vi "Inline Temporary SubVIs.vi"(8 "error in (no error)":errorcluster, 11 "Responsive Mock Class Generator in":refnum<class "Responsive Mock Class Generator.lvclass">) -> (0 "error out":errorcluster, 3 "Responsive Mock Class Generator out":refnum<class "Responsive Mock Class Generator.lvclass">)   [LabVIEW 2020, in "Responsive Mock Class Generator.lvclass"]
uses:
  Responsive Mock Class Generator.lvclass
  Responsive Mock Class Generator.lvclass/Responsive Mock Class Generator.ctl
  Framework/Responsive Mock/Append Control Value.vi
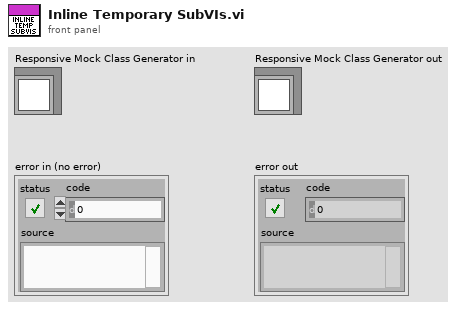
[diagram p1: front panel]
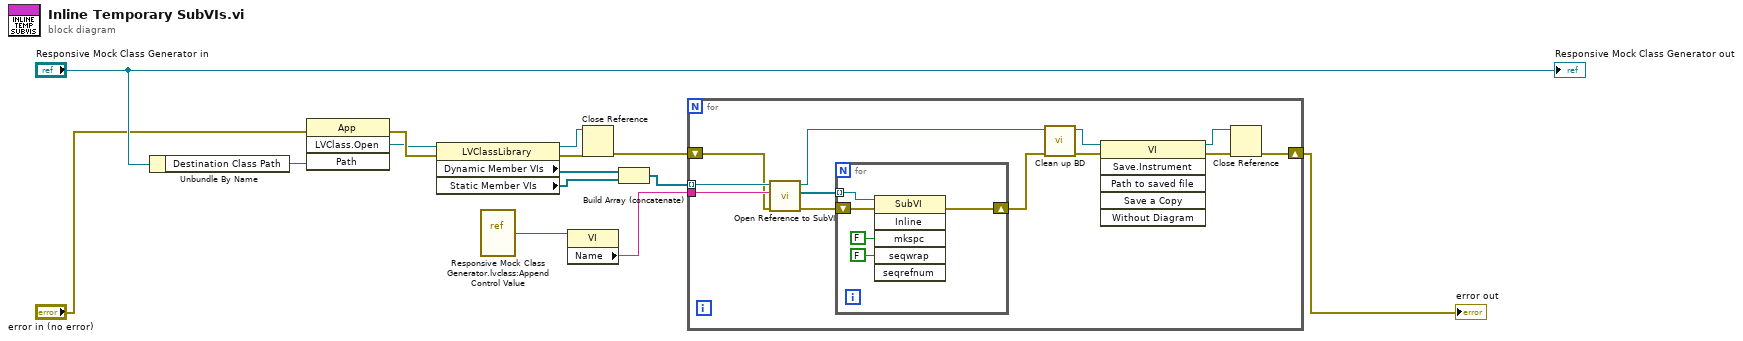
[diagram p0: block diagram]
diagram:
  n1 = Unbundle By Name("Responsive Mock Class Generator in") -> ("Destination Class Path"=w14:path)
  n2 = invoke class="App" method="LVClass.Open"(error in="error in (no error)", "Path"=w14) -> (error out=w13:errorcluster, "LVClass.Open"=w10:refnum<vi>)  [unwired: 2 in, 2 out]
  n3 = property class="LVClassLibrary"(reference=w10, error in=w13) -> (reference out=w11:refnum<vi>, error out=w12:errorcluster, "Dynamic Member VIs"=w7:refnum<vi>[], "Static Member VIs"=w6:refnum<vi>[])
  n4 = vi-ref "Responsive Mock Class Generator.lvclass:Append Control Value.vi"() -> (w5:refnum<vi>)
  n5 = property class="VI"(reference=w5) -> ("Name"=w3:string)  [unwired: 1 in, 2 out]
  n6 = Close Reference(reference=w11, error in (no error)=w12) -> (error out=w2:errorcluster)
  n7 = Build Array (concatenate)(w7, w6) -> (w4:refnum<vi>[])
  n8 = for {
    tunnel: w4 -> [w26] mode=indexing
    tunnel: w3 -> [w25]
    shift-right: [w18] -> w1
    shift-left: w2 -> [w24]
    n9 = call "Open Reference to SubVI.vi"("error in (no error)"=w24, "SubVI Name"=w25, "VI in"=w26) -> ("error out"=w23:errorcluster, "SubVIs"=w21:refnum<vi>[], "VI out"=w19:refnum<vi>)  [unwired: 6 in]
    n10 = for {
      shift-right: [w30] -> w22
      shift-left: w23 -> [w31]
      tunnel: w21 -> [w29] mode=indexing
      n11 = invoke class="SubVI" method="Inline"(reference=w29, error in=w31, "mkspc"=FALSE ("Make Space in Block Diagram"), "seqwrap"=FALSE ("Wrap in Sequence")) -> (error out=w30:errorcluster)  [unwired: 2 in, 5 out]
    }
    n12 = call "Clean up BD.vi"("error in (no error)"=w22, "VI in"=w19) -> ("error out"=w20:errorcluster, "VI out"=w16:refnum<vi>)  [unwired: 8 in]
    n13 = invoke class="VI" method="Save.Instrument"(reference=w16, error in=w20) -> (reference out=w15:refnum<vi>, error out=w17:errorcluster)  [unwired: 4 in, 4 out]
    n14 = Close Reference(reference=w15, error in (no error)=w17) -> (error out=w18:errorcluster)
  }
  "error out" <- w1
  "Responsive Mock Class Generator out" <- "Responsive Mock Class Generator in"
